vi "Button States Write.vi"(4 "error in (no error)":errorcluster, 5 "Value":bool[](array[boolean]), 6 "Container State":T3, 7 "Display State In":T1={"Buttons Displayed"=0, "Button States"=[], "Button Size"=0, "Button Style"=enum."Classic", "Active Button"=0, "Force Regen?"=FALSE, "Tip String Ref"=refnum}) -> (0 "error out":errorcluster, 3 "Display State Out":T1={"Buttons Displayed"=0, "Button States"=[], "Button Size"=0, "Button Style"=enum."Classic", "Active Button"=0, "Force Regen?"=FALSE, "Tip String Ref"=refnum})   [LabVIEW 2018, in "Toolbar.xctl"]
doc: "Sets the state of latching toolbar buttons. Transitory buttons and disabled buttons are ignored."
uses:
  Toolbar.xctl
  Button_Class/Button.lvclass
  Button_Class/Type Defs/Button Status.ctl
  <vilib>/_xctls/Container State.ctl
  <vilib>/_xctls/XControlSupport.lvlib
  Toolbar State.ctl
  Button_Class/Type Defs/Button Style.ctl
panel:
  # "Replace the Value Control below with a Control of desired type.\nDo not remove this Control or the others from the connector pane.\nDo not change the connector pane pattern.\nThe Value control should always be the third terminal from top on the input side in the connector pane."
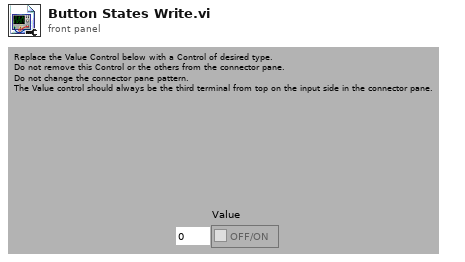
[diagram p1: front panel]
types:
  T1 = typedef "Toolbar.xctl/Toolbar State.ctl" = cluster{"Buttons Displayed":i32, "Button States":refnum<class "Button.lvclass">[], "Button Size":i32, "Button Style":T2, "Active Button":i32, "Force Regen?":bool, "Tip String Ref":refnum<vi>}
  T2 = typedef "Button.lvclass/Button Style.ctl" = enum16{"System", "Modern", "Classic", "Rounded", "Silver", "Ni Theme", "Metallic"}
  T3 = typedef "XControlSupport.lvlib/Container State.ctl" = cluster{"Indicator?":bool, "Run Mode?":bool, " Refnum":refnum<vi>}
  T4 = typedef "Button.lvclass/Button Status.ctl" = enum16{"Off", "Hover", "On", "Disabled"}
  T5 = typedef "Button.lvclass/Button Type.ctl" = enum16{"Transitory", "Latching"}
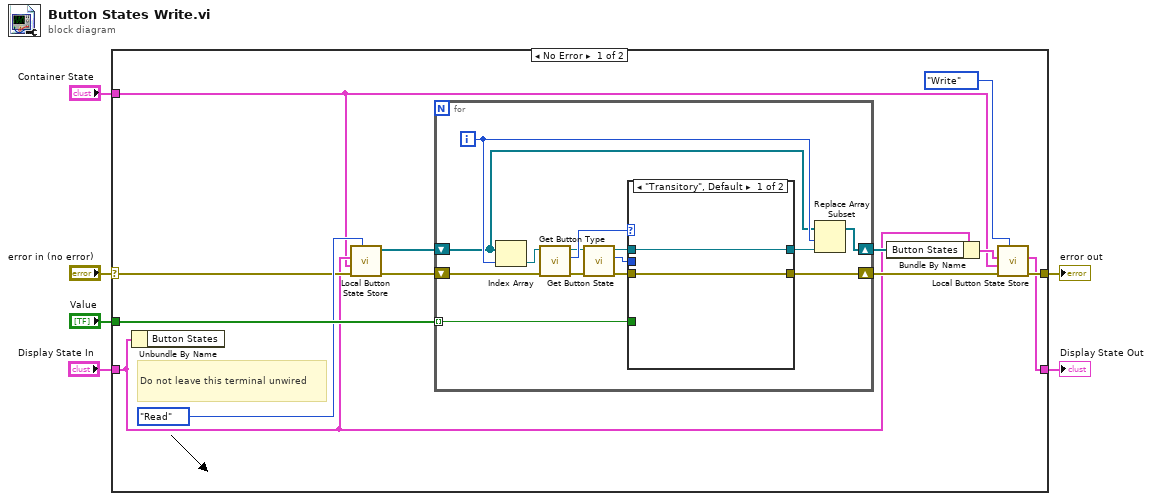
[diagram p0: block diagram]
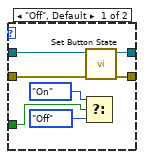
[diagram p3: hidden frame]
diagram:
  n1 = case shown="No Error" "error in (no error)" {
    selector: "error in (no error)" -> [w17 w52]
    tunnel: "Value" -> [w19 _]
    tunnel: [w13 w52] -> w4
    tunnel: "Display State In" -> [w11 w51]
    tunnel: "Container State" -> [w9 _]
    tunnel: [w8 w51] -> w1
    frame No Error {
      # "Do not leave this terminal unwired"
      n2 = Unbundle By Name(w11) -> ()  [unwired: 1 out]
      n3 = call "Local Button State Store.vi"("Operation"=enum16{"Read", "Write"}."Read", "error in (no error)"=w17, "Container State"=w9, "Display State In"=w11) -> ("error out"=w16:errorcluster, "Button States"=w7:refnum<class "Button.lvclass">[])  [unwired: 6 out]
      n4 = for {
        shift-right: [w30] -> w15
        shift-left: w7 -> [w31]
        tunnel: w19 -> [w33] mode=indexing
        shift-right: [w20] -> w14
        shift-left: w16 -> [w29]
        i -> [w32]
        n5 = Index Array(array=w31, index=w32) -> (element=w23:refnum<class "Button.lvclass">)
        n6 = call-dynamic "Get Button Type.vi"("error in (no error)"=w29, "Button in"=w23) -> ("error out"=w27:errorcluster, "Type"=w28:T5, "Button out"=w26:refnum<class "Button.lvclass">)  [unwired: 1 in, 6 out]
        n7 = call-dynamic "Get Button State.vi"("error in (no error)"=w27, "Button in"=w26) -> ("error out"=w24:errorcluster, "State"=w25:T4, "Button out"=w22:refnum<class "Button.lvclass">)  [unwired: 7 out]
        n8 = case shown="\"Transitory\", Default" w28 {
          tunnel: w25 -> [_ w41]
          tunnel: w33 -> [_ w40]
          tunnel: w24 -> [w35 w39]
          tunnel: [w34 w38] -> w21
          tunnel: [w35 w37] -> w20
          tunnel: w22 -> [w34 w36]
          frame "Transitory", Default {
          }
          frame "Latching" {
            n9 = case shown="\"Disabled\"" w41 {
              tunnel: w40 -> [w48 _]
              tunnel: w39 -> [w45 w50]
              tunnel: [w44 w49] -> w38
              tunnel: [w43 w50] -> w37
              tunnel: w36 -> [w42 w49]
              frame "Off", Default {
                n10 = Select(t=Button_Status."On", s=w48, f=Button_Status."Off" ("State")) -> ()  [unwired: 1 out]
                n11 = call-dynamic "Set Button State.vi"("error in (no error)"=w45, "Button in"=w42) -> ("error out"=w43:errorcluster, "Button out"=w44:refnum<class "Button.lvclass">)  [unwired: 1 in, 7 out]
              }
              frame "Disabled" {
              }
            }
          }
        }
        n12 = Replace Array Subset(array=w31, new element=w21, index=w32) -> (w30:refnum<class "Button.lvclass">[])
      }
      n13 = Bundle By Name(cluster=w11, "Button States"=w15) -> (w10:T1)
      n14 = call "Local Button State Store.vi"("Operation"=enum16{"Read", "Write"}."Write", "error in (no error)"=w14, "Container State"=w9, "Display State In"=w10) -> ("error out"=w13:errorcluster, "Display State Out"=w8:T1)  [unwired: 1 in, 5 out]
    }
    frame Error {
    }
  }
  "error out" <- w4
  "Display State Out" <- w1
